vi "BenchC2_DEV_v15_2.vi"() -> ()   [LabVIEW 2016]
uses:
  x64/Debug/BERTTA.dll
panel:
  out "element":bool
  out "Started:":string
  in  "SHUTDOWN":bool
  in  "MASTER CONTROL":bool
  in  "Tab Control":T1(tab)
  out "Output File":path caption="selected path"
  in  "Browse folder":path=path "" caption="start path"
  in  "Read Seq":bool
  in  "Save Seq":bool
  in  "Configuration file":path caption="Filename"
  in  "OK Button 2":bool
  out "Boolean":bool
  in  "User (initials)":string
  in  "Project name":string
  in  "Description":string
  out "PUMP1":bool
  out "Target amount":dbl
  out "Scale weight":dbl
  out "Amount now":dbl
  out "Flow rate":dbl
  out "Time to target":dbl format="%<%H:%M:%S>t"
  out "Current step":dbl
  out "Target":dbl
  out "Amount now":dbl
  out "Amount now":dbl
  out "Target":dbl
  out "Current step":dbl
  out "Time to target":dbl format="%<%H:%M:%S>t"
  out "Flow rate":dbl
  out "Amount now":dbl
  out "Scale weight":dbl
  out "Target amount":dbl
  out "PUMP2":bool
  out "Sensor OK 6":bool
  out "Sensor OK 5":bool
  out "Sensor OK 4":bool
  out "Sensor OK 3":bool
  in  "OK Button":bool
  in  "Add comment":string
  out "PUMP3":bool
  out "Target amount":dbl
  out "Scale weight":dbl
  out "Amount now":dbl
  out "Flow rate":dbl
  out "Time to target":dbl format="%<%H:%M:%S>t"
  out "Current step":dbl
  out "Target":dbl
  out "Amount now":dbl
  out "Tr":dbl
  out "Tj in":dbl
  out "Tj out":dbl
  out "T set":dbl
  out "Current step":i32
  out "RPM":dbl
  out "Torque 2":dbl
  out "Waveform Chart 5":dynamicdata(graph)
  out "Waveform Chart 6":dynamicdata(graph)
  out "Waveform Chart 7":dynamicdata(graph)
  out "Table":string[][](table)=[["14.8.2017 18.06.59", "0,000000", "417,670000", "-0,150000", "1,000000", "22,220000", "23,366837", "23,574959", "23,985852", "23,690000", "240,000000", "4,000000", "0,000000", "397,000000", "-397,000000", "1,000000"], ["14.8.2017 18.07.06", "0,000000", "417,640000", "-0,120000", "1,000000", "22,220000", "23,763115", "23,906257", "23,985694", "23,680000", "240,000000", "4,000000", "0,000000", "397,000000", "-397,000000", "1,000000"], ["14.8.2017 18.07.13", "0,000000", "417,640000", "-0,120000", "1,000000", "22,220000", "23,965922", "24,013440", "23,984906", "23,670000", "240,000000", "4,100000", "3,000000", "397,000000", "-397,000000", "1,000000"], ["14.8.2017 18.07.21", "0,000000", "417,640000", "-0,120000", "1,000000", "22,220000", "23,943860", "23,900110", "23,987113", "23,670000", "240,000000", "4,000000", "0,000000", "397,000000", "-397,000000", "1,000000"], ["14.8.2017 18.07.28", "0,000000", "417,640000", "-0,120000", "1,000000", "22,220000", "23,736328", "23,600018", "23,989004", "23,660000", "240,000000", "4,000000", "0,000000", "397,000000", "-397,000000", "1,000000"], ["14.8.2017 18.07.36", "0,000000", "417,640000", "-0,120000", "1,000000", "22,220000", "23,480910", "23,324538", "23,991053", "23,660000", "240,000000", "4,000000", "0,000000", "397,000000", "-397,000000", "1,000000"], ["14.8.2017 18.07.43", "0,000000", "417,640000", "-0,120000", "2,000000", "22,220000", "23,195579", "23,008270", "23,999093", "23,650000", "240,000000", "4,000000", "0,000000", "397,000000", "-397,000000", "1,000000"], ["14.8.2017 18.07.51", "0,000000", "417,650000", "-417,650000", "1,000000", "22,220000", "22,862541", "22,649021", "24,003979", "23,650000", "240,000000", "4,000000", "0,000000", "397,000000", "-397,000000", "2,000000"], ["14.8.2017 18.07.58", "0,000000", "417,640000", "0,010000", "1,000000", "22,220000", "22,541353", "22,354878", "24,005398", "23,650000", "240,000000", "4,000000", "0,000000", "397,000000", "-397,000000", "1,000000"], ["14.8.2017 18.08.06", "0,000000", "417,640000", "0,010000", "1,000000", "22,220000", "22,347931", "22,253738", "24,007605", "23,640000", "240,000000", "4,100000", "0,000000", "397,000000", "-397,000000", "1,000000"], ["14.8.2017 18.08.13", "0,000000", "417,640000", "0,010000", "1,000000", "22,220000", "22,329030", "22,302102", "24,006028", "23,640000", "240,000000", "4,000000", "0,000000", "395,820000", "-395,820000", "1,000000"], ["14.8.2017 18.08.20", "0,000000", "417,640000", "0,010000", "1,000000", "22,220000", "22,466849", "22,511320", "24,002403", "23,630000", "240,000000", "4,000000", "0,000000", "395,830000", "-0,010000", "1,000000"], ["14.8.2017 18.08.28", "0,000000", "417,640000", "0,010000", "1,000000", "22,220000", "22,707062", "22,835101", "24,000984", "23,620000", "240,000000", "4,000000", "0,000000", "395,830000", "-0,010000", "1,000000"], ["14.8.2017 18.08.35", "0,000000", "417,640000", "0,010000", "1,000000", "22,220000", "23,054104", "23,232979", "24,001299", "23,600000", "240,000000", "4,000000", "0,000000", "395,830000", "-0,010000", "1,000000"], ["14.8.2017 18.08.43", "0,000000", "417,640000", "0,010000", "1,000000", "22,220000", "23,412371", "23,522793", "24,002560", "23,590000", "240,000000", "4,000000", "0,000000", "395,820000", "0,000000", "1,000000"], ["14.8.2017 18.08.51", "0,000000", "417,640000", "0,010000", "1,000000", "22,220000", "23,596247", "23,656125", "24,003821", "23,580000", "240,000000", "4,000000", "0,000000", "395,820000", "0,000000", "1,000000"]]
  in  "Failsafe":dbl=20.0 format="Failsafe temperature:            %#_g"
  out "Current temp":dbl format="Current temperature S1:       %#_4g"
  out "Sensor OK":bool
  out "T external 2":dbl format="Current temperature S2:       %#_4g"
  in  "PAUSE/RUN 4":bool
  in  "Array 2":dbl[][](array[numeric])
  out "LED_3":bool
  out "LED_2":bool
  out "LED_1":bool
  out "LED_MANUAL":bool
  in  "Reset 6":bool
  in  "Manual/Ramp":bool=TRUE
  in  "Sensor selector":bool=TRUE
  in  "Tr/Tj mode selector":bool=TRUE
  in  "OK Button 3":bool
  out "Waveform Chart":dynamicdata(graph)
  out "LED STOP":bool
  out "Waveform Chart 18":dynamicdata(graph)
  in  "PAUSE/RUN 3":bool
  in  "Tube select 3":u32(ring) items=["Purple tube", "Yellow tube", " White tube"]
  in  "Reset 8":bool
  out "Led11 9":bool
  in  "?":bool
  in  "Grams / min 3":dbl
  out "RPM 3":dbl format="%_4f"
  out "Flow rate (g/min) 3":dbl
  out "Scale reading 3":dbl
  out "Step amount now 3":dbl
  out "Total amount now 3":dbl
  out "Elapsed / step 3":dbl format="%<%H:%M:%S>t"
  out "Time to target 3":dbl format="%<%H:%M:%S>t"
  out "Led5 5":bool
  out "Led4 5":bool
  out "Led3 5":bool
  out "Led2 5":bool
  out "Led1 5":bool
  in  "PumpSeq 6":dbl[][](array[numeric])=[[0.0, 0.0, 0.0, 0.0, 0.0, 0.0, 0.0, 0.0, 0.0, 0.0], [0.0, 0.0, 0.0, 0.0, 0.0, 0.0, 0.0, 0.0, 0.0, 0.0], [0.0, 0.0, 0.0, 0.0, 0.0, 0.0, 0.0, 0.0, 0.0, 0.0], [0.0, 0.0, 0.0, 0.0, 0.0, 0.0, 0.0, 0.0, 0.0, 0.0], [0.0, 0.0, 0.0, 0.0, 0.0, 0.0, 0.0, 0.0, 0.0, 0.0], [0.0, 0.0, 0.0, 0.0, 0.0, 0.0, 0.0, 0.0, 0.0, 0.0], [0.0, 0.0, 0.0, 0.0, 0.0, 0.0, 0.0, 0.0, 0.0, 0.0], [0.0, 0.0, 0.0, 0.0, 0.0, 0.0, 0.0, 0.0, 0.0, 0.0], [0.0, 0.0, 0.0, 0.0, 0.0, 0.0, 0.0, 0.0, 0.0, 0.0], [0.0, 0.0, 0.0, 0.0, 0.0, 0.0, 0.0, 0.0, 0.0, 0.0]]
  out "Led11 8":bool
  in  "PAUSE/RUN 2":bool
  in  "Tube select 2":u32(ring) items=["Purple tube", "Yellow tube", " White tube"]
  out "Led11 7":bool
  in  "?":bool
  in  "Grams / min 2":dbl
  out "RPM 2":dbl format="%_4f"
  out "Flow rate (g/min) 2":dbl
  out "Scale reading 2":dbl
  out "Step amount now 2":dbl
  out "Total amount now 2":dbl
  out "Elapsed / step 2":dbl format="%<%H:%M:%S>t"
  out "Time to target 2":dbl format="%<%H:%M:%S>t"
  out "Led5 4":bool
  out "Led4 4":bool
  out "Led3 4":bool
  out "Led2 4":bool
  out "Led1 4":bool
  in  "PumpSeq 5":dbl[][](array[numeric])=[[0.0, 0.0, 0.0, 0.0, 0.0, 0.0, 0.0, 0.0, 0.0, 0.0], [0.0, 0.0, 0.0, 0.0, 0.0, 0.0, 0.0, 0.0, 0.0, 0.0], [0.0, 0.0, 0.0, 0.0, 0.0, 0.0, 0.0, 0.0, 0.0, 0.0], [0.0, 0.0, 0.0, 0.0, 0.0, 0.0, 0.0, 0.0, 0.0, 0.0], [0.0, 0.0, 0.0, 0.0, 0.0, 0.0, 0.0, 0.0, 0.0, 0.0], [0.0, 0.0, 0.0, 0.0, 0.0, 0.0, 0.0, 0.0, 0.0, 0.0], [0.0, 0.0, 0.0, 0.0, 0.0, 0.0, 0.0, 0.0, 0.0, 0.0], [0.0, 0.0, 0.0, 0.0, 0.0, 0.0, 0.0, 0.0, 0.0, 0.0], [0.0, 0.0, 0.0, 0.0, 0.0, 0.0, 0.0, 0.0, 0.0, 0.0], [0.0, 0.0, 0.0, 0.0, 0.0, 0.0, 0.0, 0.0, 0.0, 0.0]]
  out "Led11 6":bool
  in  "Reset 7":bool
  in  "PAUSE/RUN":bool
  in  "Tube select":u32(ring) items=["Purple tube", "Yellow tube", " White tube"]
  out "Led11 5":bool
  out "RPM":dbl format="RPM                      %_4f"
  out "Flow rate (g/min)":dbl format="Flow rate               %#_g"
  out "Scale reading":dbl format="Scale reading       %#_g"
  out "Step amount now":dbl format="Step amount       %#_g"
  out "Total amount now":dbl format="Total amount      %#_g"
  out "Elapsed / step":dbl format="Elapsed / step      %<%H:%M:%S>t"
  out "Time to target":dbl format="Time to target     %<%H:%M:%S>t"
  out "Led5 3":bool
  out "Led4 3":bool
  out "Led3 3":bool
  out "Led2 3":bool
  out "Led1 3":bool
  in  "PumpSeq 4":dbl[][](array[numeric])=[[0.0, 0.0, 0.0, 0.0, 0.0, 0.0, 0.0, 0.0, 0.0, 0.0], [0.0, 0.0, 0.0, 0.0, 0.0, 0.0, 0.0, 0.0, 0.0, 0.0], [0.0, 0.0, 0.0, 0.0, 0.0, 0.0, 0.0, 0.0, 0.0, 0.0], [0.0, 0.0, 0.0, 0.0, 0.0, 0.0, 0.0, 0.0, 0.0, 0.0], [0.0, 0.0, 0.0, 0.0, 0.0, 0.0, 0.0, 0.0, 0.0, 0.0], [0.0, 0.0, 0.0, 0.0, 0.0, 0.0, 0.0, 0.0, 0.0, 0.0], [0.0, 0.0, 0.0, 0.0, 0.0, 0.0, 0.0, 0.0, 0.0, 0.0], [0.0, 0.0, 0.0, 0.0, 0.0, 0.0, 0.0, 0.0, 0.0, 0.0], [0.0, 0.0, 0.0, 0.0, 0.0, 0.0, 0.0, 0.0, 0.0, 0.0], [0.0, 0.0, 0.0, 0.0, 0.0, 0.0, 0.0, 0.0, 0.0, 0.0]]
  in  "?":bool
  in  "Grams / min":dbl format="Manual g/min:  %#_g"
  out "Led11 4":bool
  in  "Reset 5":bool
  in  "OK Button 4":bool
  out "Waveform Chart 16":dynamicdata(graph)
  in  "OK Button 5":bool
  out "Waveform Chart 17":dynamicdata(graph)
  in  "OK Button 6":bool
  in  "PAUSE/RUN 5":bool
  in  "?":bool
  in  "Scale port":dbl=5.0
  out "Waveform Chart 15":dynamicdata(graph)
  in  "OK Button 8":bool
  in  "Set RPM":i32
  in  "Remote / Manual":bool
  out "RPM":dbl
  out "Torque":dbl
  out "Waveform Chart 4":dynamicdata(graph)
  in  "OK Button 7":bool
  in  "CDAQ Temp Control":tag="cDAQ9188XT-1C3BF2FMod1"
  in  "CDAQ PAM Control":tag="cDAQ9188XT-1C3BF2FMod7"
  in  "PORT PUMP2":i32 format="PUMP 2 PORT:  %.0f"
  in  "PORT PUMP3":i32 format="PUMP 3 PORT:  %.0f"
  in  "PORT PUMP1":i32 format="PUMP 1 PORT:  %.0f"
  in  "Save PortDev":bool
  in  "LAUDA":i32 format="LAUDA PORT:  %.0f"
  in  "HEIDOLPH":i32 format="HEIDOLPH PORT:  %.0f"
  in  "SCALE1":i32 format="SCALE 1 PORT:  %.0f"
  in  "SCALE2":i32 format="SCALE 2 PORT:  %.0f"
  in  "SCALE 3":i32 format="SCALE 3 PORT:  %.0f"
  # "Temperature sensor:"
  # "Manual control:"
  # "PUMP & SCALE 1"
  # "STEP"
  # "TOTAL"
  # "PUMP & SCALE 2"
  # "STEP"
  # "TOTAL"
  # "PUMP & SCALE 3"
  # "STEP"
  # "TOTAL"
  # "STOP"
  # "MANUAL"
  # "RAMP"
  # "Temp Target       Time Target          Wait Time"
  # "g              min"
  # "g              min"
  # "g              min"
  # "PAM control"
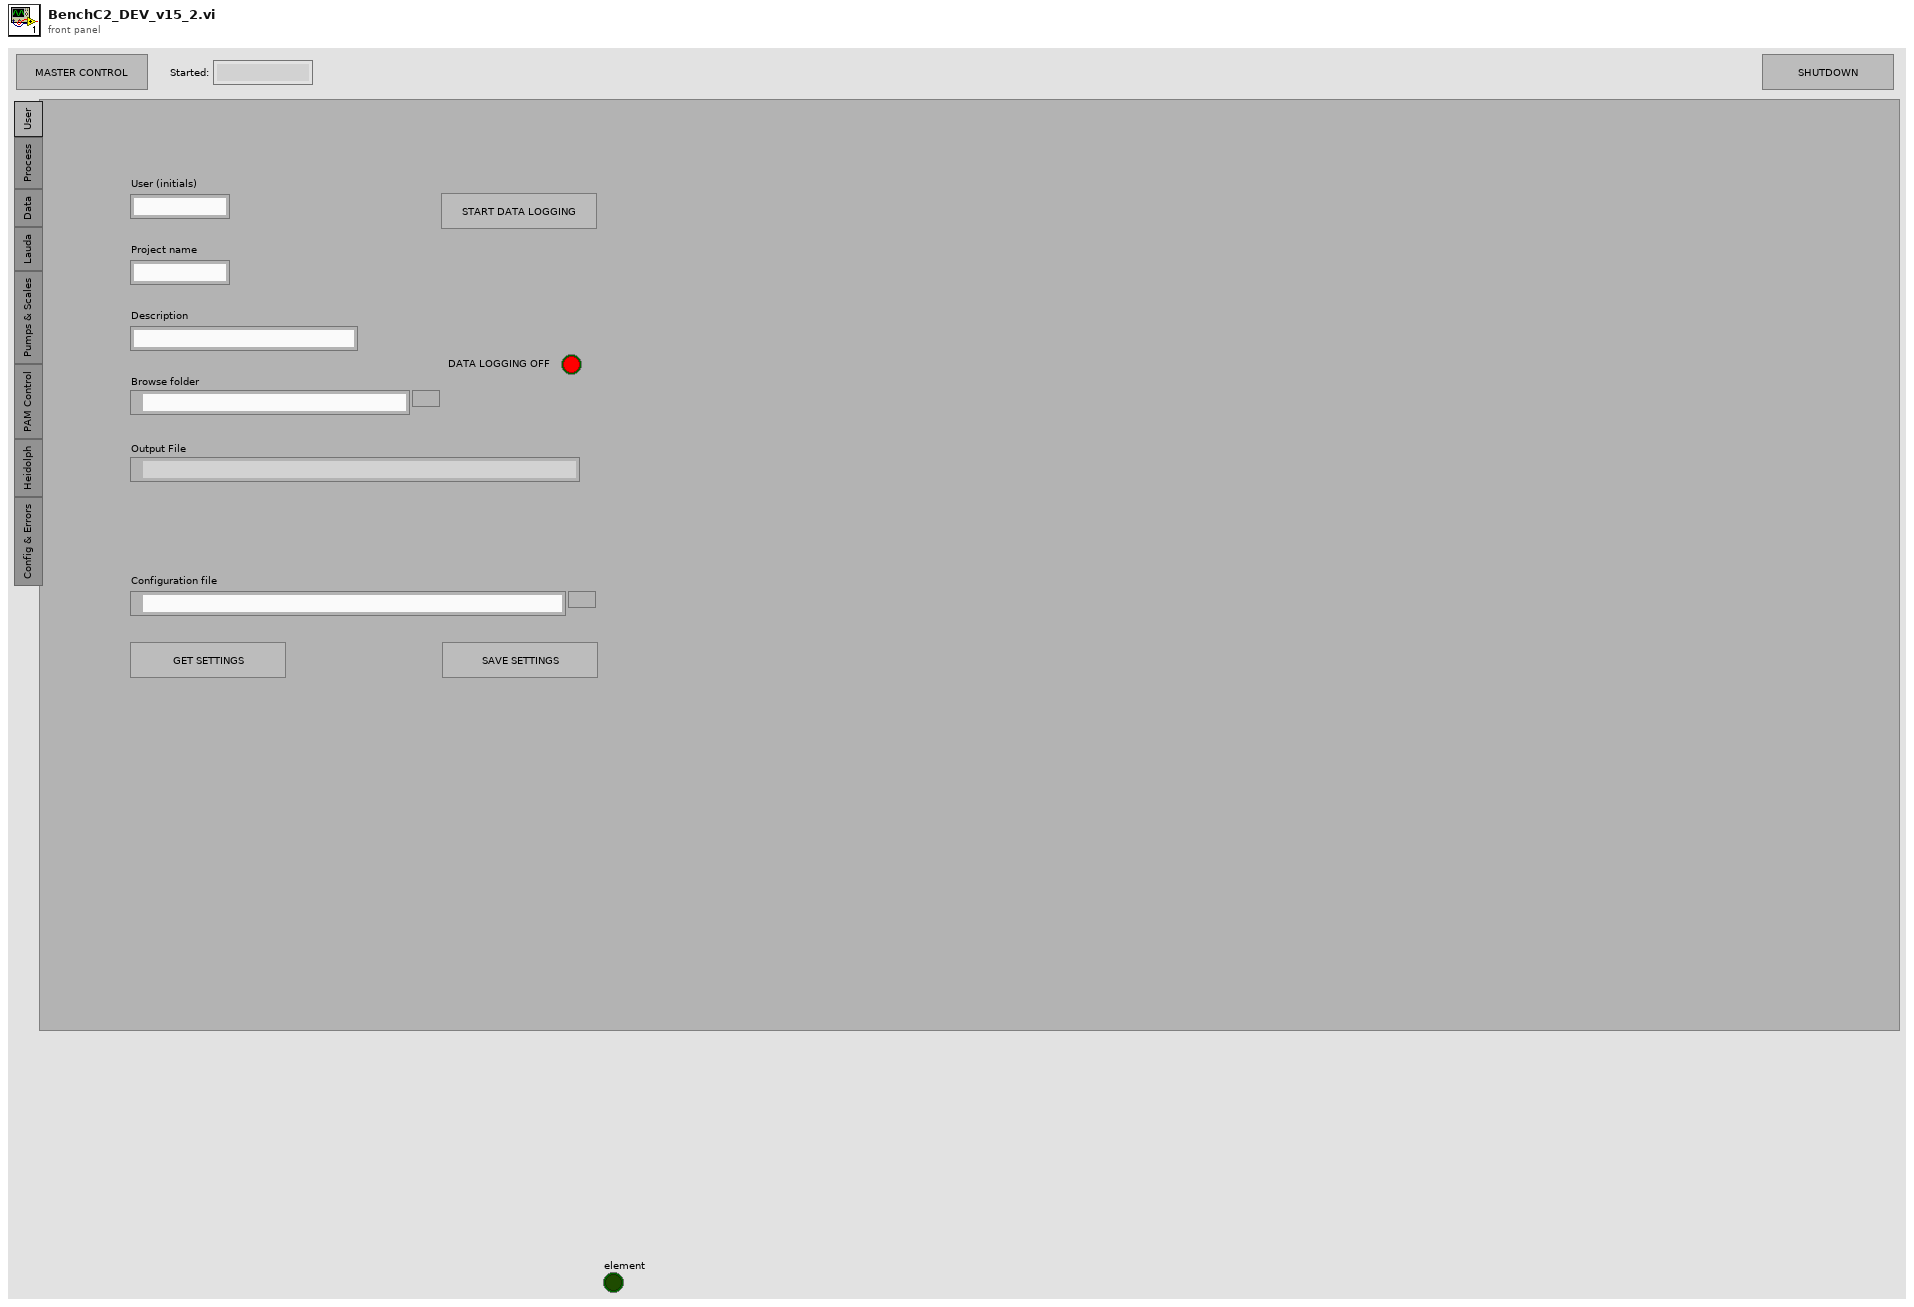
[diagram p1: front panel]
types:
  T1 = enum32{"User", "Process", "Data", "Lauda", "Pumps & Scales", "PAM Control", "Heidolph", "Config & Errors"}
diagram:
  n1 = while {
    i -> [w199]
    stop <- FALSE stop-if-true
    # "X-skaalaus puuttuu"
    # "SCALE & PUMP 1"
    # "SCALE & PUMP 3"
    n2 = Initialize Array(0.0 ("element"), 3 ("dimension size"), 3 ("dimension size")) -> (w46:dbl[][])
    n3 = Not(x="MASTER CONTROL") -> (.not. x?=w268:bool)
    n4 = Replace Array Subset(array=w46, new element="Array 2", index (row)=0, index (col)=0 ("disabled index (col)")) -> (w17:dbl[][])
    n5 = Boolean To (0,1)(Boolean=w268) -> (0, 1=w269:i16)
    n6 = for {
      N: w269 -> [_]
      n7 = Get Date/Time String(want seconds? (F)=TRUE) -> (time string=→"Started:":string)  [unwired: 2 in, 1 out]
    }
    n8 = Boolean To (0,1)(Boolean="Sensor selector") -> (0, 1=w25:i16)
    n9 = Boolean To (0,1)(Boolean="SHUTDOWN") -> (0, 1=w253:i16)
    n10 = for {
      N: w253 -> [_]
      tunnel: [w363] -> w267 mode=indexing
      i -> [w365]
      n11 = control-ref of="This VI"() -> (w368:refnum<vi>)
      n12 = invoke class="VI" method="Default Vals.Reinit All"(reference=w368) -> (reference out=w366:refnum<vi>, error out=w367:errorcluster)  [unwired: 2 in, 1 out]
      n13 = Greater?(x=w365, y=0) -> (0:w363:bool)
      n14 = Close Reference(reference=w366, error in (no error)=w367) -> ()  [unwired: 1 out]
    }
    n15 = Boolean To (0,1)(Boolean="Tr/Tj mode selector") -> (0, 1=w38:i16)
    n16 = formula code="int SensorLED1 = 0, SensorLED0 = 0, ModeLED1 = 0, ModeLED0 = 0;\nif(Sensor==1) SensorLED1 = 1;\nif(Sensor==0) SensorLED0 = 1;\nif(Tr_Tj==1) ModeLED1 = 1;\nif(Tr_Tj==0) ModeLED0 = 1;"("Tr_Tj"=w38, "Sensor"=w25) -> ("SensorLED1"=w36:i32, "SensorLED0"=w34:i32, "ModeLED1"=w18:i32, "ModeLED0"=w29:i32)
    n17 = Equal?(x=w36, y=1.0) -> (x = y?=→"Sensor OK 3":bool)
    n18 = Equal?(x=w34, y=1.0) -> (x = y?=→"Sensor OK 4":bool)
    n19 = call "MReadRS232_2.vi"("port1"="LAUDA", "dev1"=1, "port2"="LAUDA", "dev2"=2, "port3"="HEIDOLPH", "dev7"=5, "dev8"=0, "port7"="SCALE 3", "port8"=0, "dev5"=5, "port5"="SCALE1", "dev4"=4, "dev6"=5, "port6"="SCALE2", "port4"="HEIDOLPH", "dev3"=3) -> ("params"=w64:dbl[])  [unwired: 2 in, 1 out]
    n20 = call "HEI_CTRL.vi"("Set RPM"="Set RPM", "Remote / Manual"="Remote / Manual", "port3"="HEIDOLPH") -> ()  [unwired: 9 in]
    n21 = And(x="MASTER CONTROL", y="PAUSE/RUN 4") -> (x .and. y?=w67:bool)
    n22 = Index Array(array=w17, index (col)=2 ("disabled index (col)")) -> (element=w53:dbl[])  [unwired: 1 in]
    n23 = Equal?(x=w18, y=1.0) -> (x = y?=→"Sensor OK 6":bool)
    n24 = Equal?(x=w29, y=1.0) -> (x = y?=→"Sensor OK 5":bool)
    n25 = Boolean To (0,1)(Boolean=w67) -> (0, 1=w65:i16)
    n26 = Boolean To (0,1)(Boolean="Manual/Ramp") -> (0, 1=w68:i16)
    n27 = Boolean To (0,1)(Boolean="Reset 6") -> (0, 1=w70:i16)
    n28 = Build Array("LAUDA", "HEIDOLPH", "SCALE1", "SCALE2", "SCALE 3", "PORT PUMP1", "PORT PUMP2", "PORT PUMP3") -> (w3:i32[])
    n29 = feedback #1(0) -> (w251:i32)
    n30 = formula code="out = 0;\nint out2=0;\nif(in==1 ) out2 = 1;\nif(in2==1) out = 1;"("in"=w253, "in2"=w251) -> ("out"=w255:dbl, "out2"=w252:i32)
    n31 = feedback-in #1(w252) -> ()
    n32 = Index Array(array=w17, index (col)=1 ("disabled index (col)")) -> (element=w55:dbl[])  [unwired: 1 in]
    n33 = Index Array(array=w17, index (col)=0 ("disabled index (col)")) -> (element=w56:dbl[])  [unwired: 1 in]
    n34 = call "LaudaDAQ.vi"("device name"="CDAQ Temp Control") -> (1:"Tj out"=→"Tj out":dbl, "data"=w238:dynamicdata, "Sensor OK"=→"Sensor OK":bool, 4:"Tj out"=→"Tj in":dbl, "T external 2"=w26:dbl)  [unwired: 5 in, 1 out]
    "T external 2" <- w26
    n35 = Equal?(x=w255, y=1.0) -> (x = y?=w254:bool)
    n36 = Index Array(array=w267, index=0) -> (element=→"element":bool)
    n37 = call "Ramp_Lauda_v2.vi"("manual"=w68, "Tr_Tj"=w38, "S1_S2"=w25, "Tr"=w64, "T_fail"="Failsafe", "enable"=w65, "time_set"=w55, "reset"=w70, "time_wait"=w53, "T_S2"=w26, "port"="LAUDA", "T_sp"=w56) -> ("LED_1"=→"LED_1":bool, "LED_manual"=→"LED_MANUAL":bool, "LED_2"=→"LED_2":bool, "step"=w15:dbl, "LED_stop"=→"LED STOP":bool, "LED_3"=→"LED_3":bool, "setpoint"=w12:dbl, "Tr_out"=w63:dbl, "T int"=w62:dbl)  [unwired: 5 in, 2 out]
    "Tr" <- w63
    "T set" <- w12
    "Current temp" <- w63
    n38 = Stop(stop? (T)=w254) -> ()
    n39 = Boolean To (0,1)(Boolean="Save PortDev") -> (0, 1=w202:i16)
    n40 = for {
      N: w202 -> [_]
      tunnel: w3 -> [w319]
      tunnel: "Save PortDev" -> [w320]
      n41 = call "Convert to Dynamic Data"("Array"=w319) -> ("Dynamic Data Type"=w318:dynamicdata)  [unwired: 3 in]
      n42 = call "Write To Measurement File3"("Signals"=w318, "Reset"=w320) -> ()  [unwired: 15 in, 3 out]
    }
    n43 = Add(x=w15, y=1.0) -> (x+y=→"Current step":dbl)
    n44 = Less?(x=w199, y=1.0) -> (x < y?=w197:bool)
    n45 = Index Array(array=w64, index=3) -> (element=w190:dbl)
    "RPM" <- w190
    "RPM" <- w190
    n46 = Index Array(array=w64, index=2) -> (element=w192:dbl)
    n47 = Boolean To (0,1)(Boolean=w197) -> (0, 1=w198:i16)
    n48 = Divide(x=w192, y=10.0) -> (x/y=w189:dbl)
    "Torque" <- w189
    "Torque 2" <- w189
    n49 = for {
      N: w198 -> [_]
      tunnel: w197 -> [w313]
      n50 = while {
        tunnel: [w316] -> w312
        tunnel: w313 -> [w314]
        stop <- w317 stop-if-true
        n51 = call "Read From Measurement File2"("Enable"=TRUE, "Reset"=w314) -> ("Signals"=w316:dynamicdata, "EOF?"=w317:bool)  [unwired: 4 in, 4 out]
      }
      n52 = call "Convert from Dynamic Data2"("Dynamic Data Type"=w312) -> ("Array"=w298:dbl[])  [unwired: 3 in]
      n53 = Index Array(array=w298, index=0) -> (element=w305:dbl)
      n54 = Index Array(array=w298, index=1) -> (element=w304:dbl)
      n55 = Index Array(array=w298, index=2) -> (element=w303:dbl)
      n56 = Index Array(array=w298, index=3) -> (element=w302:dbl)
      n57 = Index Array(array=w298, index=4) -> (element=w301:dbl)
      n58 = Index Array(array=w298, index=5) -> (element=w295:dbl)
      n59 = Index Array(array=w298, index=6) -> (element=w297:dbl)
      n60 = Index Array(array=w298, index=7) -> (element=w296:dbl)
      n61 = property on="LAUDA" class="DigNum (strict)"("Val(Sgnl)"=w305) -> ()  [unwired: 2 in, 2 out]
      n62 = property on="HEIDOLPH" class="DigNum (strict)"("Val(Sgnl)"=w304) -> ()  [unwired: 2 in, 2 out]
      n63 = property on="SCALE1" class="DigNum (strict)"("Val(Sgnl)"=w303) -> ()  [unwired: 2 in, 2 out]
      n64 = property on="SCALE2" class="DigNum (strict)"("Val(Sgnl)"=w302) -> ()  [unwired: 2 in, 2 out]
      n65 = property on="SCALE 3" class="DigNum (strict)"("Val(Sgnl)"=w301) -> ()  [unwired: 2 in, 2 out]
      n66 = property on="PORT PUMP2" class="DigNum (strict)"("Val(Sgnl)"=w297) -> ()  [unwired: 2 in, 2 out]
      n67 = property on="PORT PUMP3" class="DigNum (strict)"("Val(Sgnl)"=w296) -> ()  [unwired: 2 in, 2 out]
      n68 = property on="PORT PUMP1" class="DigNum (strict)"("Val(Sgnl)"=w295) -> ()  [unwired: 2 in, 2 out]
    }
    n69 = Merge Signals(w190, w189) -> (w188:dynamicdata)
    "Waveform Chart 4" <- w188
    "Waveform Chart 6" <- w188
    n70 = Boolean To (0,1)(Boolean="OK Button 3") -> (0, 1=w217:i16)
    n71 = for {
      N: w217 -> [_]
      n72 = property on="Waveform Chart" class="WFChart (strict)"("History Data"=dynamicdata[] []) -> ()  [unwired: 2 in, 2 out]
    }
    n73 = Merge Signals(w12, w63, w62, w238) -> (w239:dynamicdata)
    "Waveform Chart" <- w239
    "Waveform Chart 5" <- w239
    n74 = Boolean To (0,1)(Boolean="OK Button 4") -> (0, 1=w215:i16)
    n75 = for {
      N: w215 -> [_]
      n76 = property on="Waveform Chart 18" class="WFChart (strict)"("History Data"=dynamicdata[] []) -> ()  [unwired: 2 in, 2 out]
    }
    n77 = Boolean To (0,1)(Boolean="?") -> (0, 1=w181:i16)
    n78 = Boolean To (0,1)(Boolean="PAUSE/RUN") -> (0, 1=w153:i16)
    n79 = Boolean To (0,1)(Boolean="MASTER CONTROL") -> (0, 1=w179:i16)
    n80 = Boolean To (0,1)(Boolean="Reset 5") -> (0, 1=w174:i16)
    n81 = Boolean To (0,1)(Boolean="OK Button 5") -> (0, 1=w23:i16)
    n82 = And(x=w179, y=w153) -> (x .and. y?=w178:i16)
    n83 = for {
      N: w23 -> [_]
      n84 = property on="Waveform Chart 16" class="WFChart (strict)"("History Data"=dynamicdata[] []) -> ()  [unwired: 2 in, 2 out]
    }
    n85 = Index Array(array="PumpSeq 4", index (col)=0) -> (element=w176:dbl[])  [unwired: 1 in]
    n86 = Index Array(array="PumpSeq 4", index (col)=1) -> (element=w177:dbl[])  [unwired: 1 in]
    n87 = call "PID_Flow Ctrl_2 P1.vi"("weight"=w64, "Setpoint_W"=w176, "Setpoint_T"=w177, "FrManual"="Grams / min", "enable"=w178, "manual"=w181, "reset"=w174, "tube"="Tube select") -> ("elapsed_step"=→"Elapsed / step":dbl, "total_target"=→"Target":dbl, "Setpoint_W"=→"Target amount":dbl, "LED_stop"=w152:bool, "RPM"=w175:dbl, "LED1"=→"Led1 3":bool, "LED4"=→"Led4 3":bool, "LED2"=→"Led2 3":bool, "step_amount"=→"Amount now" →"Step amount now":dbl, "LED3"=→"Led3 3":bool, "LED5"=→"Led5 3":bool, "weight"=w163:dbl, "time_to_target"=→"Time to target" →"Time to target":dbl, "PumpCTRL"=w157:dbl, "step"=→"Current step":dbl, "LED_manual"=→"Led11 5":bool, "FR"=w154:dbl)  [unwired: 3 in]
    "Flow rate" <- w154
    "Scale weight" <- w163
    "Led11 4" <- w152
    "Scale reading" <- w163
    "Flow rate (g/min)" <- w154
    "RPM" <- w175
    n88 = Merge Signals(w163, w154) -> (w24:dynamicdata)
    "Waveform Chart 18" <- w24
    n89 = Greater?(x=w157, y=70.0) -> (0:→"PUMP1":bool)
    n90 = Multiply(x=-1.0, y=w163) -> (x*y=→"Amount now" →"Total amount now":dbl)
    n91 = Boolean To (0,1)(Boolean="OK Button 6") -> (0, 1=w21:i16)
    n92 = for {
      N: w21 -> [_]
      n93 = property on="Waveform Chart 17" class="WFChart (strict)"("History Data"=dynamicdata[] []) -> ()  [unwired: 2 in, 2 out]
    }
    n94 = And(x="PAUSE/RUN", y=w152) -> (x .and. y?=w150:bool)
    n95 = feedback #2() -> (w151:bool)  [unwired: 1 in]
    n96 = feedback-in #2(w150) -> ()
    n97 = Not Equal?(x=w151, y=w150) -> (x != y?=w149:bool)
    n98 = Boolean To (0,1)(Boolean=w149) -> (0, 1=w148:i16)
    n99 = for {
      N: w148 -> [_]
      n100 = property on="PAUSE/RUN" class="Bool (strict)"("Val(Sgnl)"=FALSE ("Value (Signaling)")) -> ()  [unwired: 2 in, 2 out]
    }
    n101 = Boolean To (0,1)(Boolean="OK Button 7") -> (0, 1=w213:i16)
    n102 = for {
      N: w213 -> [_]
      n103 = property on="Waveform Chart 4" class="WFChart (strict)"("History Data"=dynamicdata[] []) -> ()  [unwired: 2 in, 2 out]
    }
    n104 = Boolean To (0,1)(Boolean="OK Button 8") -> (0, 1=w185:i16)
    n105 = for {
      N: w185 -> [_]
      n106 = property on="Waveform Chart 15" class="WFChart (strict)"("History Data"=dynamicdata[] []) -> ()  [unwired: 2 in, 2 out]
    }
    n107 = Index Array(array="PumpSeq 5", index (col)=0) -> (element=w130:dbl[])  [unwired: 1 in]
    n108 = Index Array(array="PumpSeq 5", index (col)=1) -> (element=w131:dbl[])  [unwired: 1 in]
    n109 = Boolean To (0,1)(Boolean="PAUSE/RUN 2") -> (0, 1=w146:i16)
    n110 = Boolean To (0,1)(Boolean="MASTER CONTROL") -> (0, 1=w147:i16)
    n111 = And(x=w147, y=w146) -> (x .and. y?=w145:i16)
    n112 = Boolean To (0,1)(Boolean="Reset 7") -> (0, 1=w135:i16)
    n113 = Boolean To (0,1)(Boolean="?") -> (0, 1=w137:i16)
    n114 = call "PID_Flow Ctrl_2 P2.vi"("weight"=w64, "Setpoint_W"=w130, "Setpoint_T"=w131, "FrManual"="Grams / min 2", "enable"=w145, "manual"=w137, "reset"=w135, "tube"="Tube select 2") -> ("elapsed_step"=→"Elapsed / step 2":dbl, "total_target"=→"Target":dbl, "Setpoint_W"=→"Target amount":dbl, "LED_stop"=w112:bool, "RPM"=w117:dbl, "LED1"=→"Led1 4":bool, "LED4"=→"Led4 4":bool, "LED2"=→"Led2 4":bool, "step_amount"=→"Amount now" →"Step amount now 2":dbl, "LED3"=→"Led3 4":bool, "LED5"=→"Led5 4":bool, "weight"=w79:dbl, "time_to_target"=→"Time to target" →"Time to target 2":dbl, "PumpCTRL"=w120:dbl, "step"=w125:dbl, "LED_manual"=→"Led11 7":bool, "FR"=w118:dbl)  [unwired: 3 in]
    "Scale weight" <- w79
    "Flow rate" <- w118
    "Led11 6" <- w112
    "Scale reading 2" <- w79
    "Flow rate (g/min) 2" <- w118
    "RPM 2" <- w117
    n115 = Merge Signals(w79, w118) -> (w119:dynamicdata)
    "Waveform Chart 16" <- w119
    n116 = Multiply(x=w79, y=-1.0) -> (x*y=→"Amount now" →"Total amount now 2":dbl)
    n117 = And(x="PAUSE/RUN 2", y=w112) -> (x .and. y?=w115:bool)
    n118 = Greater?(x=w120, y=70.0) -> (0:→"PUMP2":bool)
    n119 = feedback #3() -> (w116:bool)  [unwired: 1 in]
    n120 = feedback-in #3(w115) -> ()
    n121 = Not Equal?(x=w116, y=w115) -> (x != y?=w114:bool)
    n122 = Add(x=1.0, y=w125) -> (x+y=→"Current step":dbl)
    n123 = Boolean To (0,1)(Boolean=w114) -> (0, 1=w113:i16)
    n124 = for {
      N: w113 -> [_]
      n125 = property on="PAUSE/RUN 2" class="Bool (strict)"("Val(Sgnl)"=FALSE ("Value (Signaling)")) -> ()  [unwired: 2 in, 2 out]
    }
    n126 = Index Array(array="PumpSeq 6", index (col)=0) -> (element=w97:dbl[])  [unwired: 1 in]
    n127 = Index Array(array="PumpSeq 6", index (col)=1) -> (element=w98:dbl[])  [unwired: 1 in]
    n128 = Boolean To (0,1)(Boolean="MASTER CONTROL") -> (0, 1=w105:i16)
    n129 = Boolean To (0,1)(Boolean="PAUSE/RUN 3") -> (0, 1=w104:i16)
    n130 = And(x=w105, y=w104) -> (x .and. y?=w103:i16)
    n131 = Boolean To (0,1)(Boolean="?") -> (0, 1=w96:i16)
    n132 = Boolean To (0,1)(Boolean="Reset 8") -> (0, 1=w94:i16)
    n133 = call "PID_Flow Ctrl_2 P3.vi"("weight"=w64, "Setpoint_W"=w97, "Setpoint_T"=w98, "FrManual"="Grams / min 3", "enable"=w103, "manual"=w96, "reset"=w94, "tube"="Tube select 3") -> ("elapsed_step"=→"Elapsed / step 3":dbl, "total_target"=→"Target":dbl, "Setpoint_W"=→"Target amount":dbl, "LED_stop"=w72:bool, "RPM"=w77:dbl, "LED1"=→"Led1 5":bool, "LED4"=→"Led4 5":bool, "LED2"=→"Led2 5":bool, "step_amount"=→"Amount now" →"Step amount now 3":dbl, "LED3"=→"Led3 5":bool, "LED5"=→"Led5 5":bool, "weight"=w78:dbl, "time_to_target"=→"Time to target" →"Time to target 3":dbl, "PumpCTRL"=w91:dbl, "step"=w89:dbl, "LED_manual"=→"Led11 9":bool, "FR"=w83:dbl)  [unwired: 3 in]
    "Scale weight" <- w78
    "Flow rate" <- w83
    "Led11 8" <- w72
    "Scale reading 3" <- w78
    "Flow rate (g/min) 3" <- w83
    "RPM 3" <- w77
    n134 = call "MWriteRS232_1.vi"("PORT PUMP3"="PORT PUMP3", "PORT PUMP2"="PORT PUMP2", "PORT PUMP1"="PORT PUMP1", "PORT LAUDA"="LAUDA", "P3"=w77, "P2"=w117, "P1"=w175, "LAUDA"=w12) -> ()  [unwired: 4 in]
    n135 = call "Convert to Dynamic Data4"("2D Array"="PumpSeq 6") -> ("Dynamic Data Type"=w223:dynamicdata)  [unwired: 3 in]
    n136 = call "Convert to Dynamic Data3"("2D Array"="PumpSeq 5") -> ("Dynamic Data Type"=w224:dynamicdata)  [unwired: 3 in]
    n137 = call "Convert to Dynamic Data2"("2D Array"="PumpSeq 4") -> ("Dynamic Data Type"=w226:dynamicdata)  [unwired: 3 in]
    n138 = Merge Signals(w223, w224, w226) -> (w225:dynamicdata)
    n139 = Greater?(x=w91, y=70.0) -> (0:→"PUMP3":bool)
    n140 = Merge Signals(w78, w83) -> (w82:dynamicdata)
    "Waveform Chart 17" <- w82
    n141 = Add(x=1.0, y=w89) -> (x+y=→"Current step":dbl)
    n142 = Boolean To (0,1)(Boolean="Save Seq") -> (0, 1=w222:i16)
    n143 = Multiply(x=w78, y=-1.0) -> (x*y=→"Amount now" →"Total amount now 3":dbl)
    n144 = for {
      N: w222 -> [_]
      tunnel: w225 -> [w361]
      tunnel: "Configuration file" -> [w362]
      tunnel: "Save Seq" -> [w360]
      n145 = call "Write To Measurement File2"("Signals"=w361, "Reset"=w360, "Filename"=w362) -> ()  [unwired: 14 in, 3 out]
    }
    n146 = Merge Signals(w24, w119, w82) -> (w240:dynamicdata)
    n147 = Merge Signals(w163, w79, w78) -> (→"Waveform Chart 7":dynamicdata)
    n148 = And(x="MASTER CONTROL", y=w72) -> (x .and. y?=w75:bool)
    n149 = feedback #4() -> (w76:bool)  [unwired: 1 in]
    n150 = feedback-in #4(w75) -> ()
    n151 = Not Equal?(x=w76, y=w75) -> (x != y?=w74:bool)
    n152 = Boolean To (0,1)(Boolean="Read Seq") -> (0, 1=w221:i16)
    n153 = for {
      N: w221 -> [_]
      tunnel: "Configuration file" -> [w335]
      tunnel: "Read Seq" -> [w334]
      n154 = while {
        tunnel: [w359] -> w355
        tunnel: w335 -> [w358]
        tunnel: w334 -> [w356]
        stop <- w357 stop-if-true
        n155 = call "Read From Measurement File"("Filename"=w358, "Reset"=w356) -> ("Signals"=w359:dynamicdata, "EOF?"=w357:bool)  [unwired: 4 in, 4 out]
      }
      n156 = call "Convert from Dynamic Data"("Dynamic Data Type"=w355) -> ("Array"=w347:dbl[][])  [unwired: 3 in]
      n157 = Array Subset(array=w347, index (row)=20 ("index"), length (row)=10 ("length")) -> (w352:dbl[][])  [unwired: 2 in]
      n158 = Array Subset(array=w347, index (row)=10 ("index"), length (row)=10 ("length")) -> ()  [unwired: 2 in, 1 out]
      n159 = Array Subset(array=w347, index (row)=0 ("index"), length (row)=10 ("length")) -> ()  [unwired: 2 in, 1 out]
      n160 = Array Subset(array=w347, index (row)=30 ("index"), length (row)=8 ("length")) -> (w336:dbl[][])  [unwired: 2 in]
      n161 = property on="PumpSeq 4" class="Arr (strict)"("Val(Sgnl)"=w352) -> ()  [unwired: 2 in, 2 out]
      n162 = Index Array(array=w336, index (row)=2, index (col)=0 ("disabled index (col)")) -> ()  [unwired: 1 out]
      n163 = Index Array(array=w336, index (row)=4, index (col)=0 ("disabled index (col)")) -> ()  [unwired: 1 out]
      n164 = Index Array(array=w336, index (row)=0, index (col)=1 ("disabled index (col)")) -> ()  [unwired: 1 out]
      n165 = Index Array(array=w336, index (row)=1, index (col)=1 ("disabled index (col)")) -> ()  [unwired: 1 out]
    }
    n166 = Boolean To (0,1)(Boolean=w74) -> (0, 1=w73:i16)
    n167 = for {
      N: w73 -> [_]
      n168 = property on="PAUSE/RUN 3" class="Bool (strict)"("Val(Sgnl)"=FALSE ("Value (Signaling)")) -> ()  [unwired: 2 in, 2 out]
    }
    n169 = Merge Signals(w239, w240, w188) -> (w195:dynamicdata)
    n170 = call "Build Table"("Include time data"=TRUE, "Signals"=w195) -> ("Table"=w263:string[][])  [unwired: 3 in, 6 out]
    n171 = Boolean To (0,1)(Boolean="PAUSE/RUN 5") -> (0, 1=w40:i16)
    n172 = for {
      N: w40 -> [_]
      tunnel: "MASTER CONTROL" -> [w277]
      tunnel: "PAUSE/RUN 5" -> [w276]
      n173 = And(x=w276, y="?") -> (x .and. y?=w285:bool)
      n174 = dll-call lib="C:/Users/shresplab/OneDrive - Kemira Oyj/Documents/GitHub/Bertta/BERTTA/x64/Debug/BERTTA.dll" fn="mettler"("port"="Scale port", "msg"=1) -> ("return type"=w279:dbl)  [unwired: 5 in, 2 out]
      n175 = And(x=w277, y=w285) -> (x .and. y?=w282:bool)
      n176 = Initialize Array(FALSE, 1 ("dimension size")) -> (w284:bool[])
      n177 = Replace Array Subset(array=w284, new element=w282, index=0) -> (w281:bool[])
      n178 = call "Convert to Dynamic Data5"("Double"=w279) -> ("Dynamic Data Type"=→"Waveform Chart 15":dynamicdata)  [unwired: 3 in]
      n179 = call "DAQ Assistant"("data"=w281, "device name"="CDAQ PAM Control") -> ()  [unwired: 16 in, 2 out]
    }
    n180 = Delete From Array(array=w263, length=13, index (col)=0 ("index (row)")) -> (array with subset deleted=→"Table":string[][])  [unwired: 1 in, 1 out]
    n181 = call "filenameparser_09.vi"("Description"="Description", "start path"="Browse folder", "Project name"="Project name", "User (initials)"="User (initials)", "OK Button in"="OK Button 2") -> ("appended path 2"=w211:path, "appended path"=w259:path)  [unwired: 4 in, 1 out]
    "Output File" <- w211
    n182 = Boolean To (0,1)(Boolean="OK Button") -> (0, 1=w258:i16)
    n183 = for {
      N: w258 -> [_]
      tunnel: w259 -> [w326]
      w330 = " " ("string")
      n184 = property on="Add comment" class="Str"("Val(Sgnl)"="" ("Value (Signaling)")) -> ()  [unwired: 2 in, 2 out]
      n185 = Get Date/Time String(want seconds? (F)=TRUE) -> (date string=w333:string, time string=w331:string)  [unwired: 2 in]
      n186 = Concatenate Strings(w333, w330, w331, w330, "Add comment") -> (w329:string)
      n187 = feedback #5() -> (w328:string[])  [unwired: 1 in]
      n188 = Build Array (concatenate)(w328, w329) -> (w327:string[])
      n189 = feedback-in #5(w327) -> ()
      n190 = Write to Text File(file (use dialog)=w326, text=w327) -> ()  [unwired: 2 in, 3 out]
    }
    n191 = call "Header Names 4.vi"("Dynamic Data"=w195) -> ("Signals Out"=w196:dynamicdata)  [unwired: 10 in]
    n192 = call "Write To Measurement File"("Signals"=w196, "Enable"="OK Button 2", "Filename"=w211) -> ()  [unwired: 14 in, 3 out]
    "Boolean" <- "OK Button 2"
  }
